vi "Save Libraries and Projects.vi"(8 "error in":errorcluster) -> (0 "error out":errorcluster)   [LabVIEW 2021, in "Converter.lvlib"]
uses:
  Converter.lvlib
  Converter Reusables/Converter Reusables.lvlib
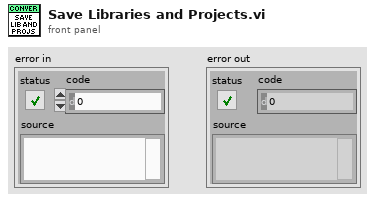
[diagram p1: front panel]
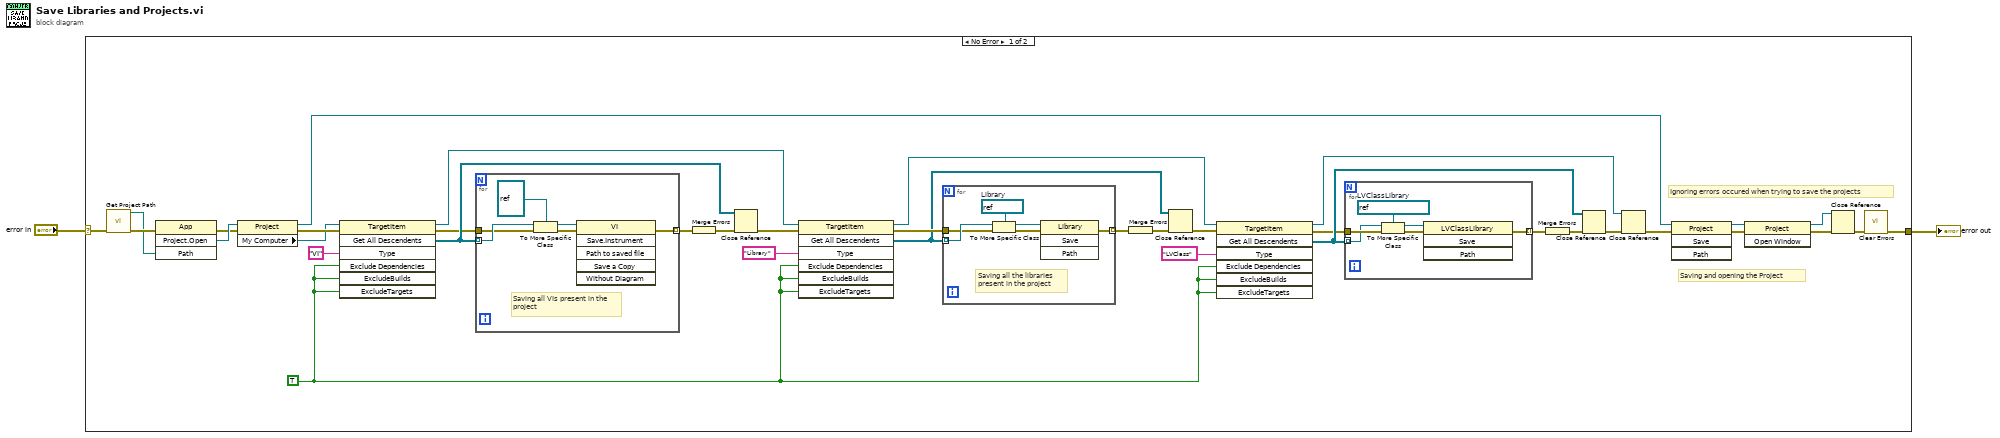
[diagram p0: block diagram]
diagram:
  n1 = case shown="No Error" "error in" {
    selector: "error in" -> [w30 w58]
    tunnel: [w10 w58] -> w2
    frame No Error {
      w6 = TRUE ("ExcludeDependencies")
      # "Saving and opening the Project"
      # "Ignoring errors occured when trying to save the projects"
      n2 = call "Get Project Path.vi"("error in"=w30) -> ("project path out"=w3:path, "error out"=w36:errorcluster)  [unwired: 13 in]
      n3 = invoke class="App" method="Project.Open"(error in=w36, "Path"=w3) -> (error out=w32:errorcluster, "Project:Open"=w34:refnum<vi>)  [unwired: 2 in, 2 out]
      n4 = property class="Project"(reference=w34, error in=w32) -> (reference out=w29:refnum<vi>, error out=w13:errorcluster, "My Computer"=w5:refnum<vi>)
      n5 = invoke class="TargetItem" method="Get All Descendents"(reference=w5, error in=w13, "Type"="VI", "Exclude Dependencies"=w6, "ExcludeBuilds"=w6, "ExcludeTargets"=w6) -> (reference out=w11:refnum<vi>, error out=w14:errorcluster, "All Descendents"=w17:refnum<vi>[])  [unwired: 1 in, 4 out]
      n6 = for {
        tunnel: w17 -> [w45] mode=indexing
        tunnel: w14 -> [w42]
        tunnel: [w43] -> w15 mode=indexing
        # "Saving all VIs present in the\nproject"
        n7 = To More Specific Class(target class=refnum<vi> refnum ("vi reference"), reference=w45, error in=w42) -> (specific class reference=w44:refnum<vi>, error out=w41:errorcluster)
        n8 = invoke class="VI" method="Save.Instrument"(reference=w44, error in=w41) -> (error out=w43:errorcluster)  [unwired: 4 in, 5 out]
      }
      n9 = Merge Errors(w15) -> (w16:errorcluster)
      n10 = Close Reference(reference=w17, error in (no error)=w16) -> (error out=w12:errorcluster)
      n11 = invoke class="TargetItem" method="Get All Descendents"(reference=w11, error in=w12, "Type"="Library", "Exclude Dependencies"=w6, "ExcludeBuilds"=w6, "ExcludeTargets"=w6) -> (reference out=w21:refnum<vi>, error out=w35:errorcluster, "All Descendents"=w27:refnum<vi>[])  [unwired: 1 in, 4 out]
      n12 = for {
        tunnel: w27 -> [w57] mode=indexing
        tunnel: w35 -> [w54]
        tunnel: [w55] -> w33 mode=indexing
        w56 = refnum<vi> refnum  # Library
        # "Saving all the libraries \npresent in the project"
        n13 = To More Specific Class(target class=w56, reference=w57, error in=w54) -> (specific class reference=w53:refnum<vi>, error out=w52:errorcluster)
        n14 = invoke class="Library" method="Save"(reference=w53, error in=w52) -> (error out=w55:errorcluster)  [unwired: 2 in, 3 out]
      }
      n15 = Merge Errors(w33) -> (w28:errorcluster)
      n16 = Close Reference(reference=w27, error in (no error)=w28) -> (error out=w22:errorcluster)
      n17 = invoke class="TargetItem" method="Get All Descendents"(reference=w21, error in=w22, "Type"="LVClass", "Exclude Dependencies"=w6, "ExcludeBuilds"=w6, "ExcludeTargets"=w6) -> (reference out=w20:refnum<vi>, error out=w23:errorcluster, "All Descendents"=w26:refnum<vi>[])  [unwired: 1 in, 4 out]
      n18 = for {
        tunnel: w26 -> [w46] mode=indexing
        tunnel: w23 -> [w48]
        tunnel: [w49] -> w24 mode=indexing
        w51 = refnum<vi> refnum  # LVClassLibrary
        n19 = To More Specific Class(target class=w51, reference=w46, error in=w48) -> (specific class reference=w50:refnum<vi>, error out=w47:errorcluster)
        n20 = invoke class="LVClassLibrary" method="Save"(reference=w50, error in=w47) -> (error out=w49:errorcluster)  [unwired: 2 in, 3 out]
      }
      n21 = Merge Errors(w24) -> (w25:errorcluster)
      n22 = Close Reference(reference=w26, error in (no error)=w25) -> (error out=w19:errorcluster)
      n23 = Close Reference(reference=w20, error in (no error)=w19) -> (error out=w18:errorcluster)
      n24 = invoke class="Project" method="Save"(reference=w29, error in=w18) -> (reference out=w37:refnum<vi>, error out=w38:errorcluster)  [unwired: 2 in, 2 out]
      n25 = invoke class="Project" method="Open Window"(reference=w37, error in=w38) -> (reference out=w9:refnum<vi>, error out=w39:errorcluster)  [unwired: 1 in, 1 out]
      n26 = Close Reference(reference=w9, error in (no error)=w39) -> (error out=w31:errorcluster)
      n27 = call <vilib>:"Clear Errors.vi"("error in (no error)"=w31) -> ("error out"=w10:errorcluster)  [unwired: 5 in, 1 out]
    }
    frame Error {
    }
  }
  "error out" <- w2
